vi "Core-CatchAndClearError.vi"(8 "Err-I":errorcluster, 11 "ErrQ-I":refnum<queue>) -> (0 "Err-O":errorcluster)   [LabVIEW 2021]
doc: "Catch and Clear the Error\nIf an error happened or user want to exit application(indicated by user error code:9999),\nEnqueue error information to error queue then clear error.\n\nNotes:\n- It is very important to make sure the error were cleared \nso that each loop can be continousely run."
panel:
  # "Inputs"
  # "Outputs"
  # ":: Modularized Parallism Templete ::\n- Catch Error -\nby: HighTech <HighTechYoung@yahoo.com>\nCopyright (C) 2010, Vision Technologies All Rights Reserved"
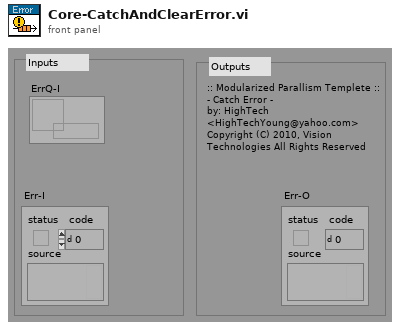
[diagram p1: front panel]
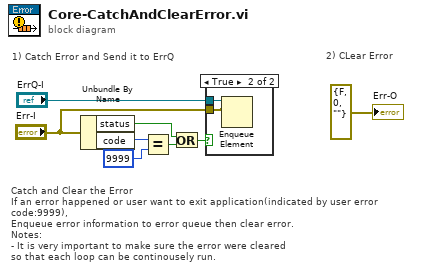
[diagram p0: block diagram]
diagram:
  # "2) CLear Error"
  # "1) Catch Error and Send it to ErrQ"
  # "Catch and Clear the Error\nIf an error happened or user want to exit application(indicated by user error code:9999),\nEnqueue error information to error queue then clear error.\nNotes:\n- It is very important to make sure the error were cleared \nso that each loop can be continousely run."
  n1 = Unbundle By Name("Err-I") -> ("status"=w6:bool, "code"=w8:i32)
  n2 = Equal?(x=w8, y=9999) -> (x = y?=w7:bool)
  n3 = Or(x=w6, y=w7) -> (x .or. y?=w4:bool)
  n4 = case shown="True" w4 {
    tunnel: "ErrQ-I" -> [_ w10]
    tunnel: "Err-I" -> [_ w9]
    frame False {
    }
    frame True {
      n5 = Enqueue Element(queue=w10, element=w9) -> ()  [unwired: 1 in, 4 out]
    }
  }
  "Err-O" <- errorcluster {"status"=FALSE, "code"=0, "source"=""} ("Err-O")
